vi "Script Execution.vi"() -> ()   [LabVIEW 2011]
uses:
  Classes/WorkorderHandler/Software/DataStructures/WorkorderHandler_ObjectReference.ctl
  <vilib>/Utility/miscctls.llb/LVRowAndColumnTypeDef.ctl
  Strict Type Controls/Settings Operation.ctl
  <vilib>/DAQmx/write.llb/DAQmx Write (Digital U32 1Chan 1Samp).vi
  <vilib>/DAQmx/create/channels.llb/DAQmx Create Channel (DO-Digital Output).vi
  <vilib>/DAQmx/miscellaneous.llb/DAQmx Fill In Error Info.vi
  <vilib>/Instr/_visa.llb/VISA Configure Serial Port (Instr).vi
panel:
  out "error out":errorcluster
  in  "error in (no error)":errorcluster
  out "Quit":bool
  in  "Heading":string="Regulator Test Bench With IEM Testing"
  in  "Edit":bool
  in  "Run":bool
  out "Order Number":string
  in  "Open":bool
  out "Bad Boards":u32
  out "Good Boards":u32
  out "result":bool=TRUE
  in  "Part Number":string
  out "Test Time":string
  in  "Result":i32(listbox)
  out "Regulator Voltage":dbl[](graph)
  out "DF Voltage":dbl[](graph)
  out "File Name":string
  out "Progress":u8(slide) scale=0.0..100.0
  # "App Designed For:"
  # "Web: www.jambhekar.com\nEmail: tushar@jambhekar.com\nCell: +919970168164"
  # "App Designed By:"
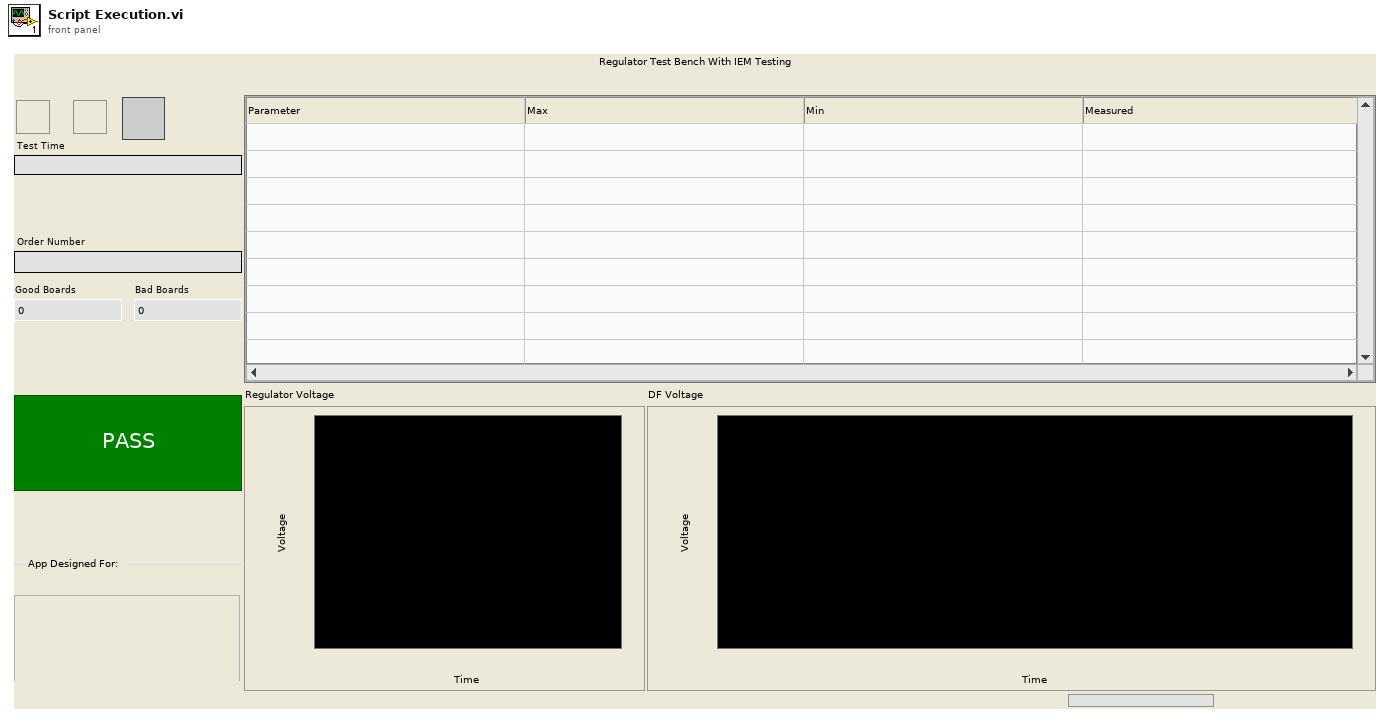
[diagram p1: front panel]
types:
  T1 = typedef "WorkorderHandler_ObjectReference.ctl" = refnum<k1>
  T2 = cluster{"Script":string[][], "Id":i32, "FailedOnce":bool, "Result":bool, "PassRef":refnum<file>, "FailRef":refnum<file>, "ScrName":string, "WORef":T1}
  T3 = enum32{"invalid app kind", "Development System", "Run Time System", "Student Edition", "Embedded LabVIEW", "Evaluation", "Custom"}
  T4 = typedef "Settings Operation.ctl" = enum8{"Get Value", "Set Value", "Read File", "Write File", "Write Stored Value"}
  T5 = typedef "LVRowAndColumnTypeDef.ctl" = cluster{"Row":i32, "Column":i32}
  T6 = enum32{"Invalid", "Standard", "Closed", "Hidden", "Minimized", "Maximized"}
  T7 = enum8{"Enabled", "Disabled", "Disabled and Grayed Out"}
  T8 = typedef "DispSettings.ctl" = cluster{"ShowDF":bool, "ShowPartNo":bool, "DF Pos":i32}
  T9 = cluster{"Port":refnum<visa-resource-name>, "baud rate":u32, "data bits":u16, "stop bits":u16, "parity":enum16{"None", "Odd", "Even", "Mark", "Space"}, "flow control":u16}
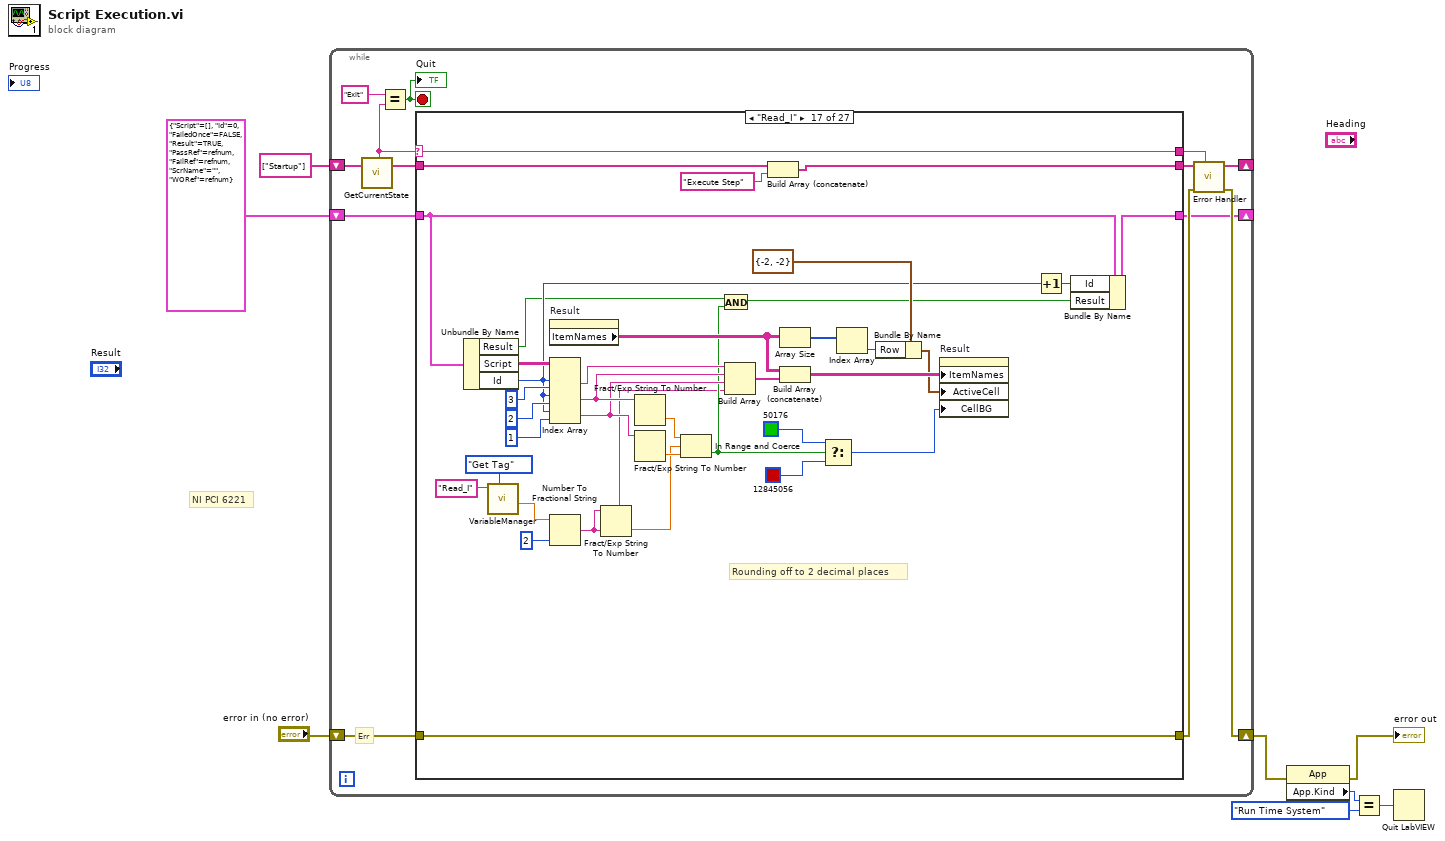
[diagram p0: block diagram]
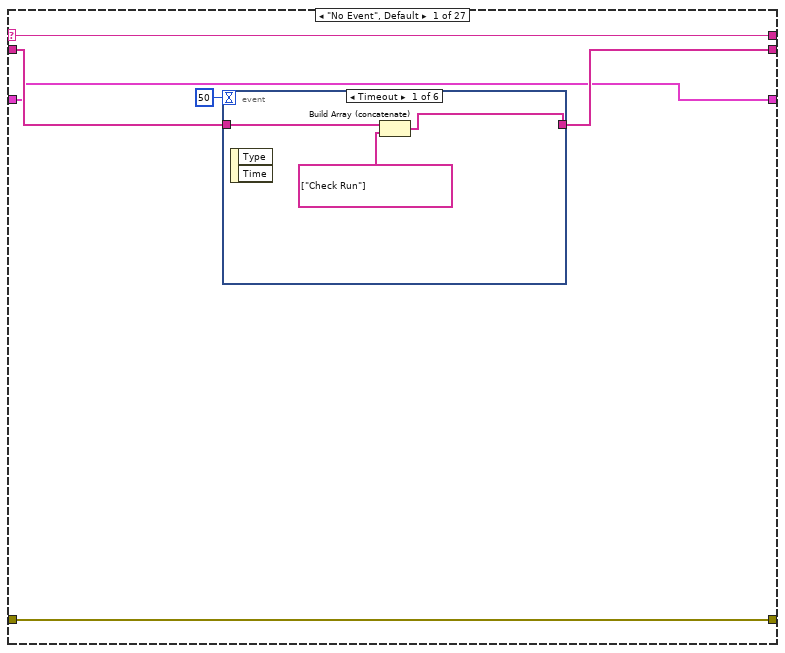
[diagram p2: hidden frame]
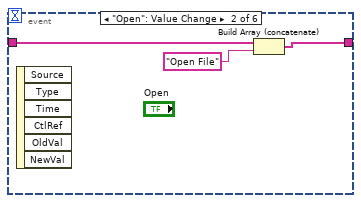
[diagram p3: hidden frame]
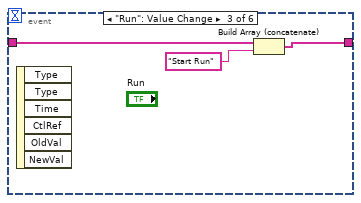
[diagram p4: hidden frame]
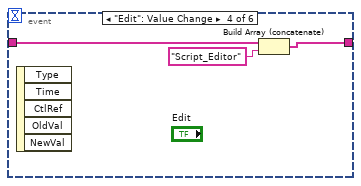
[diagram p5: hidden frame]
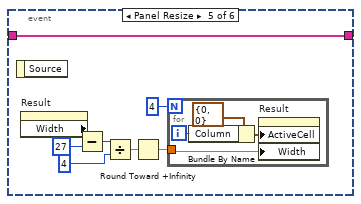
[diagram p6: hidden frame]
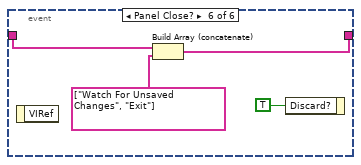
[diagram p7: hidden frame]
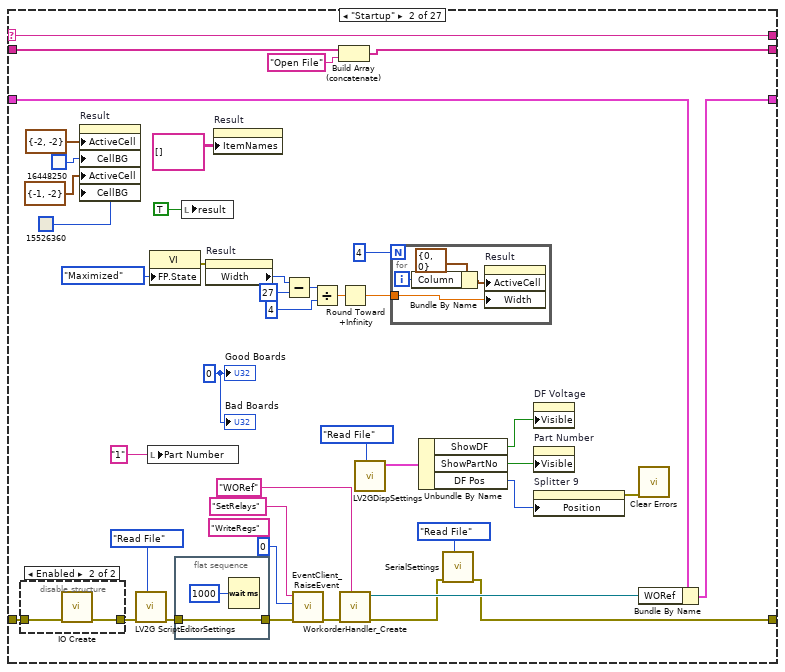
[diagram p8: hidden frame]
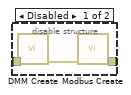
[diagram p9: hidden frame]
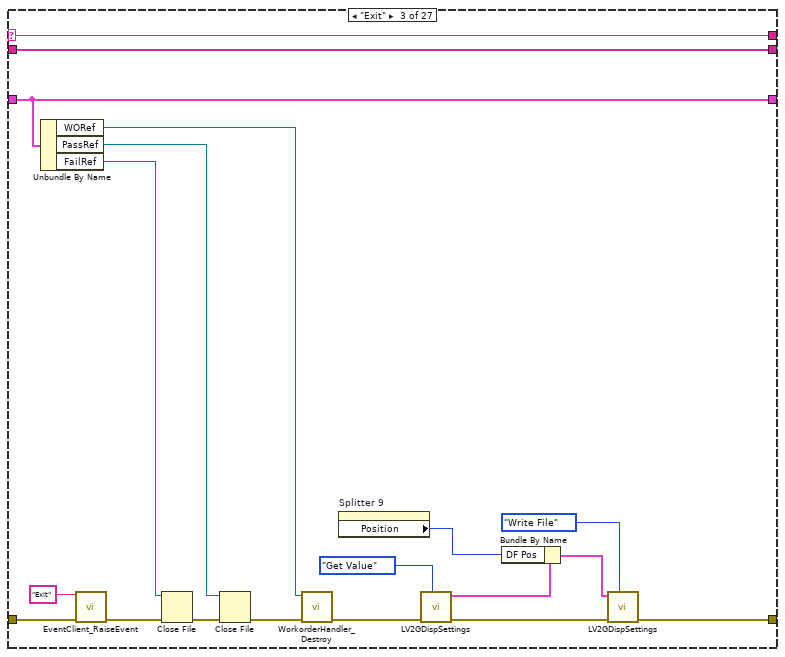
[diagram p10: hidden frame]
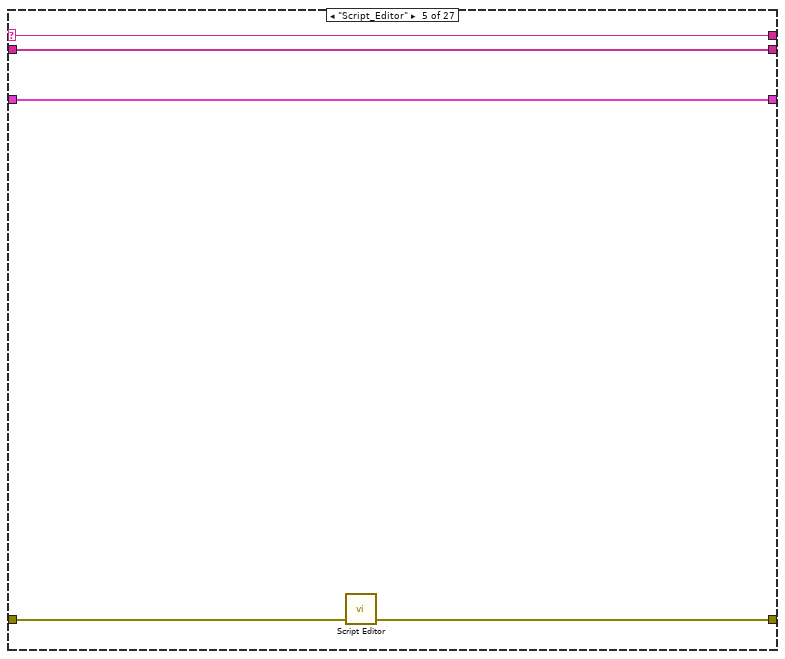
[diagram p12: hidden frame]
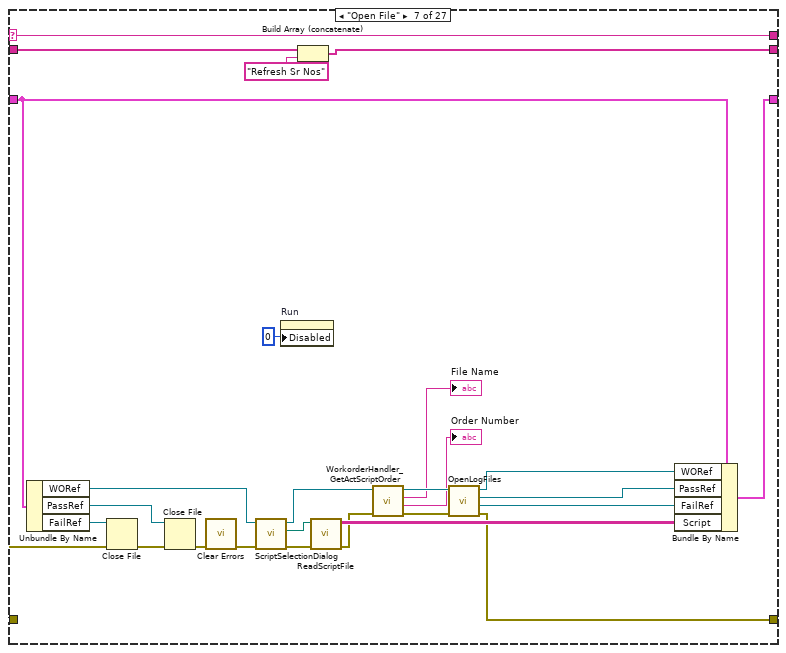
[diagram p14: hidden frame]
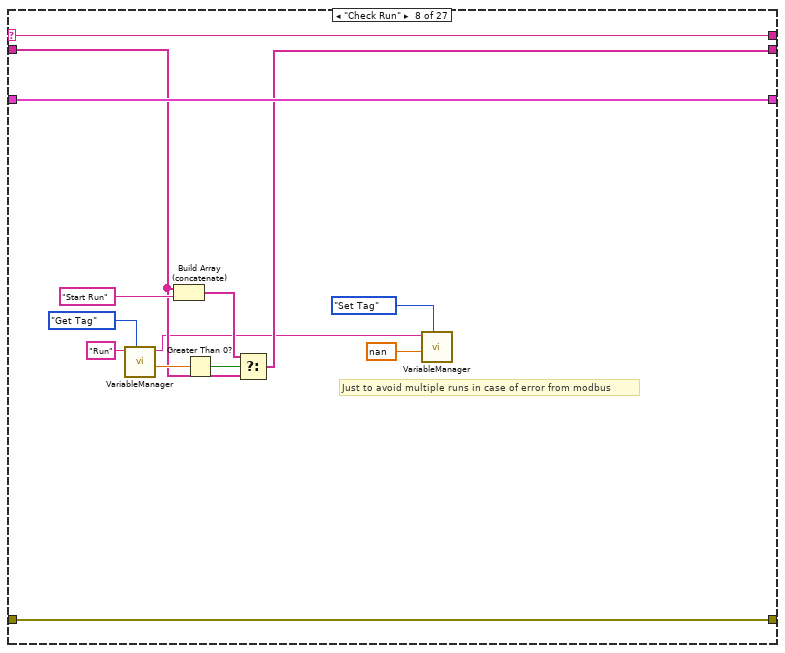
[diagram p15: hidden frame]
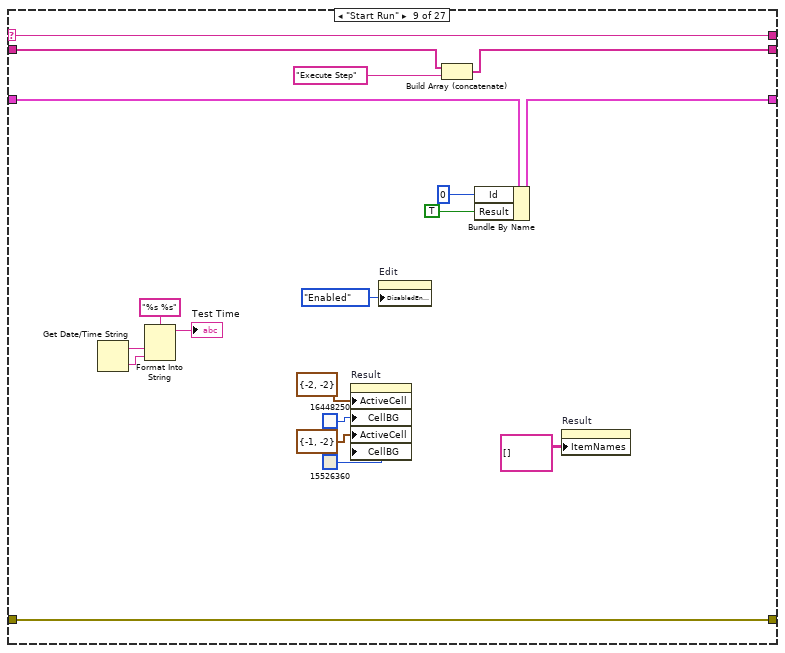
[diagram p16: hidden frame]
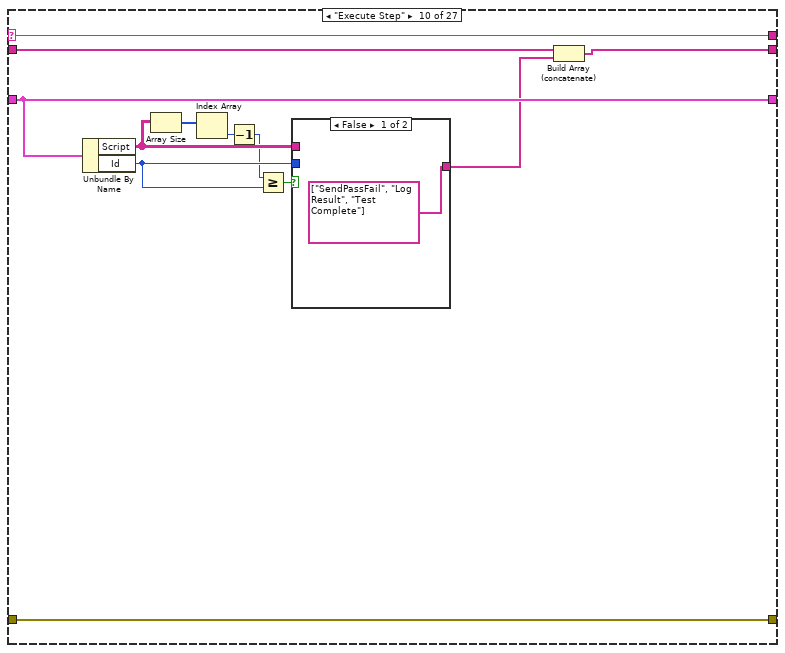
[diagram p17: hidden frame]
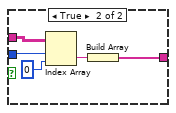
[diagram p18: hidden frame]
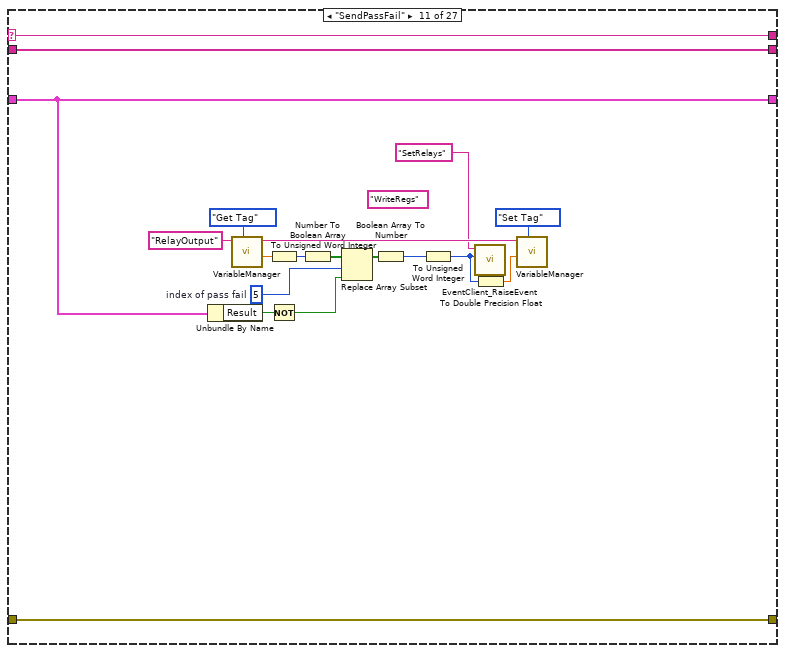
[diagram p19: hidden frame]
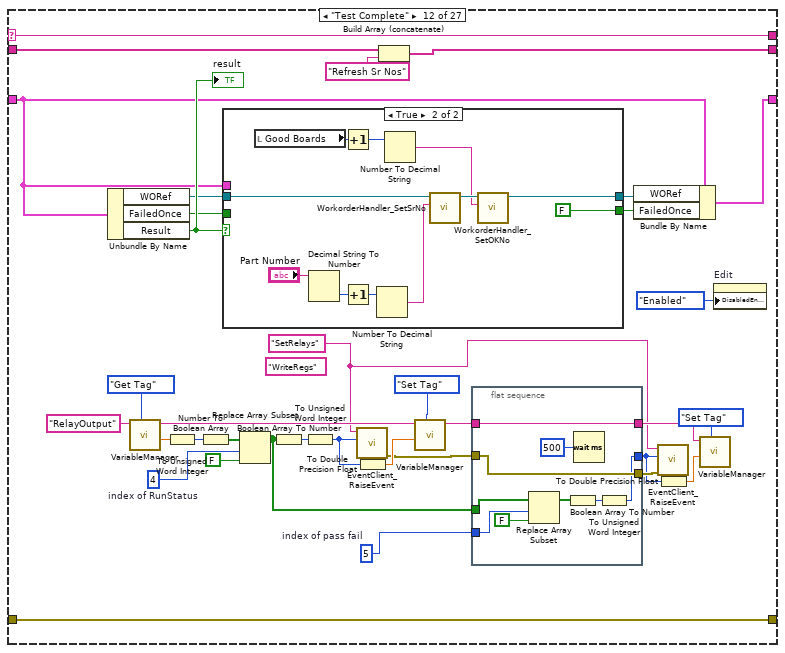
[diagram p20: hidden frame]
diagram:
  # "NI PCI 6221"
  n1 = while {
    shift-right: [w16] -> _
    shift-left: string[] ["Startup"] ("State Array Out") -> [w21]
    shift-right: [w13] -> w2
    shift-left: "error in (no error)" -> [w17]
    shift-right: [w10] -> _
    shift-left: T2 {"Script"=[], "Id"=0, "FailedOnce"=FALSE, "Result"=TRUE, "PassRef"=refnum, "FailRef"=refnum, "ScrName"="", "WORef"=refnum} ("Cluster") -> [w9]
    stop <- w18 stop-if-true
    # "Err"
    n2 = call "GetCurrentState.vi"("State Array In"=w21) -> ("Current State"=w11:string, "State Array Out"=w20:string[])  [unwired: 1 in, 16 out]
    n3 = Equal?(x="Exit", y=w11) -> (x = y?=w18:bool)
    "Quit" <- w18
    n4 = case shown="\"Read_I\"" w11 {
      selector: w11 -> [w27 w97 w126 w129 w136 w138 w167 w180 w199 w211 w236 w271 w329 w337 w374 w411 w448 w484 w521 w558 w572 w599 w628 w639 w655 w680 w684]
      tunnel: w20 -> [w23 w81 w127 w131 w135 w140 w142 w172 w190 w210 w235 w242 w328 w335 w372 w409 w446 w482 w519 w556 w570 w597 w626 w629 w646 w679 w683]
      tunnel: [w24 w80 w127 w131 w135 w140 w141 w171 w189 w209 w235 w241 w328 w335 w371 w408 w445 w481 w518 w555 w569 w596 w625 w629 w645 w679 w683] -> w15
      tunnel: [w26 w57 w114 w130 w132 w139 w144 w181 w200 w212 w237 w272 w314 w338 w375 w412 w449 w485 w522 w559 w573 w574 w610 w630 w648 w678 errorcluster {"status"=FALSE, "code"=0, "source"=""} ("error in (no error)")] -> w12
      tunnel: w17 -> [w26 w86 w125 w130 w133 w139 w158 w181 w200 w212 w237 w272 w315 w338 w375 w412 w449 w485 w522 w559 w573 w575 w611 w631 w649 w678 _]
      tunnel: [w27 w97 w126 w129 w136 w138 w167 w180 w199 w211 w236 w271 w329 w337 w374 w411 w448 w484 w521 w558 w572 w599 w628 w639 w655 w680 w684] -> w14
      tunnel: [w22 w67 w123 w128 w134 w137 w166 w175 w193 w206 w221 w266 w319 w336 w345 w382 w419 w458 w495 w532 w563 w590 w620 w636 w643 w677 w681] -> w10
      tunnel: w9 -> [w22 w68 w123 w128 w134 w137 w159 w175 w194 w206 w221 w267 w319 w336 w346 w383 w420 w459 w496 w533 w564 w591 w621 w636 w644 w677 w681]
      frame "No Event", Default {
        n5 = event shown="[0] Timeout" {
          selector: _ -> [_ _ _ _ _ _]
          dyn-events: _ -> [_ _ _ _ _ _]
          timeout: 50 -> [_ _ _ _ _ _]
          tunnel: w23 -> [w29 w33 w36 w39 w42 w54]
          tunnel: [w28 w32 w35 w38 w42 w52] -> w24
          event Timeout {
            n6 = event-data() -> ()  [unwired: 3 out]
            n7 = Build Array (concatenate)(w29, string[] ["Check Run"] ("State Array Out")) -> (w28:string[])
          }
          event "Open": Value Change {
            n8 = event-data() -> ()  [unwired: 7 out]
            n9 = Build Array (concatenate)(w33, "Open File" ("x")) -> (w32:string[])
          }
          event "Run": Value Change {
            n10 = event-data() -> ()  [unwired: 7 out]
            n11 = Build Array (concatenate)(w36, "Start Run" ("x")) -> (w35:string[])
          }
          event "Edit": Value Change {
            n12 = event-data() -> ()  [unwired: 6 out]
            n13 = Build Array (concatenate)(w39, "Script_Editor") -> (w38:string[])
          }
          event Panel Resize {
            n14 = event-data() -> ()  [unwired: 2 out]
            n15 = property on="Result" class="MCListbox (strict)"() -> ("Width"=w40:u32)  [unwired: 2 in, 2 out]
            n16 = Subtract(x=w40, y=u32 27) -> (x-y=w44:u32)
            n17 = Divide(x=w44, y=u32 4) -> (x/y=w46:dbl)
            n18 = Round Toward +Infinity(x=w46) -> (ceil(x): smallest int >= x=w47:dbl)
            n19 = for {
              N: 4 -> [_]
              tunnel: w47 -> [w48]
              i -> [w50]
              n20 = Bundle By Name(cluster=cluster{"Row":i32, "Column":i32} {"Row"=0, "Column"=0} ("Active Cell:Active Cell"), "Column"=w50) -> (w49:cluster{"Row":i32, "Column":i32})
              n21 = property on="Result" class="MCListbox (strict)"("ActiveCell"=w49, "Width"=w48) -> ()  [unwired: 2 in, 2 out]
            }
          }
          event Panel Close? {
            n22 = event-data() -> ()  [unwired: 2 out]
            n23 = Build Array (concatenate)(w54, string[] ["Watch For Unsaved Changes", "Exit"] ("State Array Out")) -> (w52:string[])
            n24 = event-data("Discard?"=TRUE) -> ()  [unwired: 1 in, 1 out]
          }
        }
      }
      frame "Startup" {
        w75 = u32 0 ("Good Boards")
        (unwired) "WriteRegs" ("Tag")
        n25 = disable-structure shown="Enabled" {
          disable-tunnel: w86 -> [w99 w102]
          disable-tunnel: [w98 w101] -> w85
          frame Disabled {
            n26 = call "DMM Create.vi"("error in (no error)"=w99) -> ("error out"=w100:errorcluster)  [unwired: 10 out]
            n27 = call "Modbus Create.vi"("error in (no error)"=w100) -> ("error out"=w98:errorcluster)  [unwired: 10 out]
          }
          frame Enabled {
            n28 = call "IO Create.vi"("error in (no error)"=w102) -> ("error out"=w101:errorcluster)  [unwired: 10 in]
          }
        }
        n29 = property on="Result" class="MCListbox (strict)"("ActiveCell"=T5 {"Row"=-2, "Column"=-2} ("Active Cell:Active Cell"), "CellBG"=u32 16448250, "ActiveCell"=T5 {"Row"=-1, "Column"=-2} ("Active Cell:Active Cell"), "CellBG"=u32 15526360 ("Color Box")) -> ()  [unwired: 2 in, 2 out]
        n30 = call "LV2G ScriptEditorSettings.vi"("Operation"=Settings_Operation."Read File", "error in (no error)"=w85) -> ("error out"=w77:errorcluster)  [unwired: 1 in, 8 out]
        n31 = local write "Part Number"("1" ("Part Number")) -> ()
        n32 = property class="VI"("FP.State"=T6."Maximized" ("Front Panel Window:State")) -> (error out=w87:errorcluster)  [unwired: 2 in, 1 out]
        n33 = flat-sequence {
          tunnel: [w103] -> w76
          tunnel: w77 -> [w103]
          frame #0 {
            n34 = Wait (ms)(milliseconds to wait=u32 1000) -> ()  [unwired: 1 out]
          }
        }
        n35 = local write "result"(TRUE ("result")) -> ()
        n36 = property on="Result" class="MCListbox (strict)"(error in=w87) -> ("Width"=w90:u32)  [unwired: 1 in, 2 out]
        n37 = property on="Result" class="MCListbox (strict)"("ItemNames"=string[][] [] ("Item Names")) -> ()  [unwired: 2 in, 2 out]
        n38 = Subtract(x=w90, y=u32 27) -> (x-y=w92:u32)
        n39 = call "EventClient_RaiseEvent.vi"("error in (no error)"=w76, "Data"=u16 0, "Event"="SetRelays" ("Tag")) -> ("error out"=w71:errorcluster)  [unwired: 1 in, 7 out]
        n40 = Divide(x=w92, y=u32 4) -> (x/y=w94:dbl)
        n41 = Build Array (concatenate)(w81, "Open File" ("String")) -> (w80:string[])
        n42 = Round Toward +Infinity(x=w94) -> (ceil(x): smallest int >= x=w95:dbl)
        n43 = call "WorkorderHandler_Create.vi"("object name (unnamed)"="WORef", "error in (no error)"=w71) -> ("error out"=w58:errorcluster, "reference"=w69:T1)  [unwired: 8 out]
        n44 = call "LV2GDispSettings.vi"("Operation"=Settings_Operation."Read File") -> ("DispSettings out"=w65:T8)  [unwired: 2 in, 8 out]
        n45 = for {
          N: 4 -> [_]
          tunnel: w95 -> [w105]
          i -> [w107]
          n46 = Bundle By Name(cluster=cluster{"Row":i32, "Column":i32} {"Row"=0, "Column"=0} ("Active Cell:Active Cell"), "Column"=w107) -> (w106:cluster{"Row":i32, "Column":i32})
          n47 = property on="Result" class="MCListbox (strict)"("ActiveCell"=w106, "Width"=w105) -> ()  [unwired: 2 in, 2 out]
        }
        n48 = Unbundle By Name(w65) -> ("ShowDF"=w63:bool, "ShowPartNo"=w62:bool, "DF Pos"=w64:i32)
        n49 = call "SerialSettings.vi"("Operation"=Settings_Operation."Read File", "error in (no error)"=w58) -> ("error out"=w57:errorcluster)  [unwired: 8 in, 1 out]
        n50 = property on="DF Voltage" class="WFGraph (strict)"("Visible"=w63) -> ()  [unwired: 2 in, 2 out]
        n51 = property on="Part Number" class="Str"("Visible"=w62) -> ()  [unwired: 2 in, 2 out]
        n52 = property on="Splitter 9" class="Splitter"("Position"=w64) -> (error out=w61:errorcluster)  [unwired: 2 in, 1 out]
        n53 = call <vilib>:"Clear Errors.vi"("error in (no error)"=w61) -> ()  [unwired: 7 out]
        n54 = Bundle By Name(cluster=w68, "WORef"=w69) -> (w67:T2)
        "Good Boards" <- w75
        "Bad Boards" <- w75
      }
      frame "Exit" {
        n55 = Unbundle By Name(w123) -> ("WORef"=w117:T1, "PassRef"=w119:refnum<file>, "FailRef"=w120:refnum<file>)
        n56 = call "EventClient_RaiseEvent.vi"("error in (no error)"=w125, "Event"="Exit" ("x")) -> ("error out"=w122:errorcluster)  [unwired: 2 in, 7 out]
        n57 = Close File(refnum=w120, error in=w122) -> (error out=w121:errorcluster)  [unwired: 1 out]
        n58 = Close File(refnum=w119, error in=w121) -> (error out=w118:errorcluster)  [unwired: 1 out]
        n59 = call "WorkorderHandler_Destroy.vi"("error in (no error)"=w118, "reference"=w117) -> ("error out"=w116:errorcluster)  [unwired: 9 out]
        n60 = property on="Splitter 9" class="Splitter"() -> ("Position"=w109:i32)  [unwired: 2 in, 2 out]
        n61 = call "LV2GDispSettings.vi"("Operation"=Settings_Operation."Get Value", "error in (no error)"=w116) -> ("error out"=w115:errorcluster, "DispSettings out"=w111:T8)  [unwired: 1 in, 7 out]
        n62 = Bundle By Name(cluster=w111, "DF Pos"=w109) -> (w110:T8)
        n63 = call "LV2GDispSettings.vi"("Operation"=Settings_Operation."Write File", "error in (no error)"=w115, "DispSettings"=w110) -> ("error out"=w114:errorcluster)  [unwired: 8 out]
      }
      frame "---------------Below are UI Events---------------" {
      }
      frame "Script_Editor" {
        n64 = call "Script Editor.vi"("error in (no error)"=w133) -> ("error out"=w132:errorcluster)  [unwired: 4 in]
      }
      frame "---------------Below are Subroutine states---------------" {
      }
      frame "Open File" {
        n65 = Unbundle By Name(w159) -> ("WORef"=w155:T1, "PassRef"=w161:refnum<file>, "FailRef"=w160:refnum<file>)
        n66 = Close File(refnum=w160, error in=w158) -> (error out=w162:errorcluster)  [unwired: 1 out]
        n67 = Close File(refnum=w161, error in=w162) -> (error out=w157:errorcluster)  [unwired: 1 out]
        n68 = call <vilib>:"Clear Errors.vi"("error in (no error)"=w157) -> ("error out"=w156:errorcluster)  [unwired: 6 out]
        n69 = call "ScriptSelectionDialog.vi"("error in (no error)"=w156, "WORef"=w155) -> ("error out"=w163:errorcluster, "Path"=w154:path, "WORef Out"=w151:T1)  [unwired: 7 out]
        n70 = property on="Run" class="Bool"("Disabled"=u8 0) -> ()  [unwired: 2 in, 2 out]
        n71 = Build Array (concatenate)(w142, "Refresh Sr Nos" ("x")) -> (w141:string[])
        n72 = call "ReadScriptFile.vi"("error in (no error)"=w163, "File"=w154) -> ("error out"=w149:errorcluster, "Script"=w164:string[][])  [unwired: 1 in, 7 out]
        n73 = call "WorkorderHandler_GetActScriptOrder.vi"("error in (no error)"=w149, "reference"=w151) -> ("error out"=w148:errorcluster, "Order"=→"Order Number":string, "Script"=→"File Name":string, "duplicate reference"=w150:T1)  [unwired: 6 out]
        n74 = call "OpenLogFiles.vi"("error in (no error)"=w148, "WORef"=w150) -> ("error out"=w144:errorcluster, "FailRef"=w153:refnum<file>, "PassRef"=w152:refnum<file>, "WORef Out"=w145:T1)  [unwired: 6 out]
        n75 = Bundle By Name(cluster=w159, "WORef"=w145, "PassRef"=w152, "FailRef"=w153, "Script"=w164) -> (w166:T2)
      }
      frame "Check Run" {
        # "Just to avoid multiple runs in case of error from modbus"
        n76 = call "VariableManager.vi"("Operation"=enum16{"Get Tag", "Set Tag"}."Get Tag", "Tag"="Run") -> ("Value out"=w177:dbl, "Tag Out"=w169:string)  [unwired: 1 in, 7 out]
        n77 = Build Array (concatenate)(w172, "Start Run" ("x")) -> (w173:string[])
        n78 = Greater Than 0?(x=w177) -> (x > 0?=w176:bool)
        n79 = Select(t=w173, s=w176, f=w172) -> (s? t:f=w171:string[])
        n80 = call "VariableManager.vi"("Operation"=enum16{"Get Tag", "Set Tag"}."Set Tag", "Value"=nan, "Tag"=w169) -> ()  [unwired: 9 out]
      }
      frame "Start Run" {
        n81 = Get Date/Time String() -> (date string=w198:string, time string=w197:string)  [unwired: 3 out]
        n82 = Format Into String(format string="%s %s", w198, w197) -> (resulting string=→"Test Time":string)  [unwired: 2 in, 1 out]
        n83 = property on="Result" class="MCListbox (strict)"("ActiveCell"=T5 {"Row"=-2, "Column"=-2} ("Active Cell:Active Cell"), "CellBG"=u32 16448250, "ActiveCell"=T5 {"Row"=-1, "Column"=-2} ("Active Cell:Active Cell"), "CellBG"=u32 15526360 ("Color Box")) -> ()  [unwired: 2 in, 2 out]
        n84 = property on="Edit" class="Bool"("DisabledEnum"=T7."Enabled" ("Disabled")) -> ()  [unwired: 2 in, 2 out]
        n85 = Build Array (concatenate)(w190, "Execute Step" ("x")) -> (w189:string[])
        n86 = Bundle By Name(cluster=w194, "Id"=0, "Result"=TRUE) -> (w193:T2)
        n87 = property on="Result" class="MCListbox (strict)"("ItemNames"=string[][] [] ("Item Names")) -> ()  [unwired: 2 in, 2 out]
      }
      frame "Execute Step" {
        n88 = Unbundle By Name(w206) -> ("Script"=w204:string[][], "Id"=w203:i32)
        n89 = Array Size(array=w204) -> (size(s)=w208:i32[])
        n90 = Index Array(array=w208) -> (element=w207:i32)  [unwired: 1 in]
        n91 = Decrement(x=w207) -> (x-1=w201:i32)
        n92 = Greater Or Equal?(x=w201, y=w203) -> (x >= y?=w205:bool)
        n93 = case shown="False" w205 {
          tunnel: w204 -> [_ w218]
          tunnel: w203 -> [_ w217]
          tunnel: [string[] ["SendPassFail", "Log Result", "Test Complete"] ("State Array Out") w214] -> w202
          frame False {
          }
          frame True {
            n94 = Index Array(array=w218, index (row)=w217, index (col)=0 ("disabled index (col)")) -> (element=w215:string)
            n95 = Build Array(w215) -> (w214:string[])
          }
        }
        n96 = Build Array (concatenate)(w210, w202) -> (w209:string[])
      }
      frame "SendPassFail" {
        w227 = 5  # index of pass fail
        (unwired) "WriteRegs" ("Tag")
        n97 = Unbundle By Name(w221) -> ("Result"=w220:bool)
        n98 = call "VariableManager.vi"("Operation"=enum16{"Get Tag", "Set Tag"}."Get Tag", "Tag"="RelayOutput") -> ("Value out"=w232:dbl, "Tag Out"=w222:string)  [unwired: 1 in, 7 out]
        n99 = To Unsigned Word Integer(number=w232) -> (unsigned 16bit integer=w231:u16)
        n100 = Not(x=w220) -> (.not. x?=w226:bool)
        n101 = Number To Boolean Array(number=w231) -> (Boolean array=w230:bool[])
        n102 = Replace Array Subset(array=w230, new element=w226, index=w227) -> (w229:bool[])
        n103 = Boolean Array To Number(Boolean array=w229) -> (number=w228:u32)
        n104 = To Unsigned Word Integer(number=w228) -> (unsigned 16bit integer=w224:u16)
        n105 = call "EventClient_RaiseEvent.vi"("Data"=w224, "Event"="SetRelays" ("Tag")) -> ()  [unwired: 2 in, 8 out]
        n106 = To Double Precision Float(number=w224) -> (double precision float=w223:dbl)
        n107 = call "VariableManager.vi"("Operation"=enum16{"Get Tag", "Set Tag"}."Set Tag", "Value"=w223, "Tag"=w222) -> ()  [unwired: 9 out]
      }
      frame "Test Complete" {
        w238 = "SetRelays" ("Tag")
        w252 = 5  # index of pass fail
        w259 = 4  # index of RunStatus
        (unwired) "WriteRegs" ("Tag")
        n108 = Unbundle By Name(w267) -> ("WORef"=w244:T1, "FailedOnce"=w268:bool, "Result"=w269:bool)
        "result" <- w269
        n109 = call "VariableManager.vi"("Operation"=enum16{"Get Tag", "Set Tag"}."Get Tag", "Tag"="RelayOutput") -> ("Value out"=w263:dbl, "Tag Out"=w256:string)  [unwired: 1 in, 7 out]
        n110 = To Unsigned Word Integer(number=w263) -> (unsigned 16bit integer=w262:u16)
        n111 = Number To Boolean Array(number=w262) -> (Boolean array=w261:bool[])
        n112 = case shown="True" w269 {
          tunnel: w267 -> [_ _]
          tunnel: [w285 FALSE] -> w270
          tunnel: w268 -> [w284 _]
          tunnel: w244 -> [w283 w298]
          tunnel: [w282 w294] -> w243
          frame False {
            n113 = case shown="True" w284 {
              tunnel: [TRUE FALSE] -> w285
              tunnel: w283 -> [w286 w291]
              tunnel: [w286 w288] -> w282
              frame False {
              }
              frame True {
                n114 = local read "Bad Boards"() -> (w293:u32)
                n115 = Increment(x=w293) -> (x+1=w290:u32)
                n116 = Number To Decimal String(number=w290) -> (decimal integer string=w289:string)  [unwired: 1 out]
                n117 = call "WorkorderHandler_SetBadNo.vi"("BadNo"=w289, "reference"=w291) -> ("duplicate reference"=w288:T1)  [unwired: 1 in, 8 out]
              }
            }
          }
          frame True {
            n118 = local read "Good Boards"() -> (w301:u32)
            n119 = Decimal String To Number(string="Part Number") -> (number=w304:i32)  [unwired: 3 out]
            n120 = Increment(x=w301) -> (x+1=w296:u32)
            n121 = Increment(x=w304) -> (x+1=w303:i32)
            n122 = Number To Decimal String(number=w303) -> (decimal integer string=w299:string)  [unwired: 1 out]
            n123 = Number To Decimal String(number=w296) -> (decimal integer string=w295:string)  [unwired: 1 out]
            n124 = call "WorkorderHandler_SetSrNo.vi"("SrNo"=w299, "reference"=w298) -> ("duplicate reference"=w297:T1)  [unwired: 1 in, 8 out]
            n125 = call "WorkorderHandler_SetOKNo.vi"("OKNo"=w295, "reference"=w297) -> ("duplicate reference"=w294:T1)  [unwired: 1 in, 8 out]
          }
        }
        n126 = Replace Array Subset(array=w261, new element=FALSE ("new element/subarray"), index=w259) -> (w253:bool[])
        n127 = Boolean Array To Number(Boolean array=w253) -> (number=w260:u32)
        n128 = To Unsigned Word Integer(number=w260) -> (unsigned 16bit integer=w254:u16)
        n129 = call "EventClient_RaiseEvent.vi"("Data"=w254, "Event"=w238) -> ("error out"=w249:errorcluster)  [unwired: 2 in, 7 out]
        n130 = To Double Precision Float(number=w254) -> (double precision float=w257:dbl)
        n131 = Build Array (concatenate)(w242, "Refresh Sr Nos" ("x")) -> (w241:string[])
        n132 = call "VariableManager.vi"("Operation"=enum16{"Get Tag", "Set Tag"}."Set Tag", "Value"=w257, "Tag"=w256) -> ("Tag Out"=w245:string)  [unwired: 8 out]
        n133 = flat-sequence {
          tunnel: w253 -> [w280]
          tunnel: w252 -> [w279]
          tunnel: w249 -> [w276]
          tunnel: [w276] -> w248
          tunnel: [w275] -> w247
          tunnel: [w274] -> w246
          tunnel: w245 -> [w274]
          frame #0 {
            n134 = Replace Array Subset(array=w280, new element=FALSE ("new element/subarray"), index=w279) -> (w277:bool[])
            n135 = Boolean Array To Number(Boolean array=w277) -> (number=w278:u32)
            n136 = Wait (ms)(milliseconds to wait=u32 500) -> ()  [unwired: 1 out]
            n137 = To Unsigned Word Integer(number=w278) -> (unsigned 16bit integer=w275:u16)
          }
        }
        n138 = Bundle By Name(cluster=w267, "WORef"=w243, "FailedOnce"=w270) -> (w266:T2)
        n139 = call "EventClient_RaiseEvent.vi"("error in (no error)"=w248, "Data"=w247, "Event"=w238) -> ()  [unwired: 1 in, 8 out]
        n140 = To Double Precision Float(number=w247) -> (double precision float=w251:dbl)
        n141 = call "VariableManager.vi"("Operation"=enum16{"Get Tag", "Set Tag"}."Set Tag", "Value"=w251, "Tag"=w246) -> ()  [unwired: 9 out]
        n142 = property on="Edit" class="Bool"("DisabledEnum"=T7."Enabled" ("Disabled")) -> ()  [unwired: 2 in, 2 out]
      }
      frame "Log Result" {
        n143 = local read "Good Boards"() -> (w309:u32)
        n144 = local read "Bad Boards"() -> (w308:u32)
        n145 = Unbundle By Name(w319) -> ("PassRef"=w318:refnum<file>, "Result"=w310:bool, "FailRef"=w317:refnum<file>, "FailedOnce"=w311:bool)
        n146 = Or(x=w310, y=w311) -> (x .or. y?=w312:bool)
        n147 = Select(t=w318, s=w310, f=w317) -> (s? t:f=w316:refnum<file>)
        n148 = Select(t=w309, s=w310, f=w308) -> (s? t:f=w307:u32)
        n149 = Increment(x=w307) -> (x+1=w305:u32)
        n150 = Number To Decimal String(number=w305) -> (decimal integer string=w306:string)  [unwired: 1 out]
        n151 = local read "Test Time"() -> (w313:string)
        n152 = property on="Result" class="MCListbox (strict)"() -> ("ItemNames"=w327:string[][])  [unwired: 2 in, 2 out]
        n153 = Index Array(array=w327, index (col)=3 ("disabled index (col)")) -> (element=w321:string[])  [unwired: 1 in]
        n154 = Build Array (concatenate)(w306, w313, w321) -> (w320:string[])
        n155 = Array To Spreadsheet String(array=w320, 3:"%s" ("format string")) -> (spreadsheet string=w323:string)  [unwired: 1 out]
        n156 = Concatenate Strings(w323, "\r\n") -> (w322:string)
        n157 = case shown="True" w312 {
          tunnel: w322 -> [_ w334]
          tunnel: w316 -> [_ w333]
          tunnel: w315 -> [w330 w332]
          tunnel: [w330 w331] -> w314
          frame False {
          }
          frame True {
            n158 = Write to Text File(file (use dialog)=w333, text=w334, error in=w332) -> (error out=w331:errorcluster)  [unwired: 3 out]
          }
        }
      }
      frame "---------------Below are Step states---------------" {
      }
      frame "Read DMM" {
        # "Rounding off to 2 decimal places"
        n159 = Unbundle By Name(w346) -> ("Result"=w343:bool, "Script"=w370:string[][], "Id"=w347:i32)
        n160 = call "VariableManager.vi"("Operation"=enum16{"Get Tag", "Set Tag"}."Get Tag", "Tag"="DMM") -> ("Value out"=w359:dbl)  [unwired: 1 in, 8 out]
        n161 = property on="Result" class="MCListbox (strict)"() -> ("ItemNames"=w356:string[][])  [unwired: 2 in, 2 out]
        n162 = Index Array(array=w370, index (row) #1=w347, index (col) #1=3 ("disabled index (col)"), index (row) #2=w347, index (col) #2=2 ("disabled index (col)"), index (row) #3=w347, index (col) #3=1 ("disabled index (col)")) -> (element #1=w365:string, element #2=w363:string, element #3=w362:string)
        n163 = Number To Fractional String(number=w359, precision (6)=i16 2) -> (F-format string=w340:string)  [unwired: 2 out]
        n164 = Fract/Exp String To Number(string=w340) -> (number=w339:dbl)  [unwired: 4 out]
        n165 = Fract/Exp String To Number(string=w363) -> (number=w361:dbl)  [unwired: 4 out]
        n166 = Fract/Exp String To Number(string=w362) -> (number=w360:dbl)  [unwired: 4 out]
        n167 = In Range and Coerce(upper limit=w361, x=w339, lower limit=w360) -> (In Range?=w344:bool)  [unwired: 1 out]
        n168 = And(x=w343, y=w344) -> (x .and. y?=w342:bool)
        n169 = Build Array(w365, w363, w362, w340) -> (w358:string[])
        n170 = Build Array (concatenate)(w372, "Execute Step" ("x")) -> (w371:string[])
        n171 = Array Size(array=w356) -> (size(s)=w355:i32[])
        n172 = Build Array (concatenate)(w356, w358) -> (w357:string[][])
        n173 = Select(t=u32 50176, s=w344, f=u32 12845056) -> (s? t:f=w349:u32)
        n174 = Index Array(array=w355) -> (element=w353:i32)  [unwired: 1 in]
        n175 = Bundle By Name(cluster=T5 {"Row"=-2, "Column"=-2} ("Active Cell:Active Cell"), "Row"=w353) -> (w352:T5)
        n176 = property on="Result" class="MCListbox (strict)"("ItemNames"=w357, "ActiveCell"=w352, "CellBG"=w349) -> ()  [unwired: 2 in, 2 out]
        n177 = Increment(x=w347) -> (x+1=w348:i32)
        n178 = Bundle By Name(cluster=w346, "Id"=w348, "Result"=w342) -> (w345:T2)
      }
      frame "Read_V" {
        # "Rounding off to 2 decimal places"
        n179 = Unbundle By Name(w383) -> ("Result"=w380:bool, "Script"=w407:string[][], "Id"=w384:i32)
        n180 = call "VariableManager.vi"("Operation"=enum16{"Get Tag", "Set Tag"}."Get Tag", "Tag"="Read_V") -> ("Value out"=w396:dbl)  [unwired: 1 in, 8 out]
        n181 = property on="Result" class="MCListbox (strict)"() -> ("ItemNames"=w393:string[][])  [unwired: 2 in, 2 out]
        n182 = Index Array(array=w407, index (row) #1=w384, index (col) #1=3 ("disabled index (col)"), index (row) #2=w384, index (col) #2=2 ("disabled index (col)"), index (row) #3=w384, index (col) #3=1 ("disabled index (col)")) -> (element #1=w402:string, element #2=w400:string, element #3=w399:string)
        n183 = Number To Fractional String(number=w396, precision (6)=i16 2) -> (F-format string=w377:string)  [unwired: 2 out]
        n184 = Fract/Exp String To Number(string=w377) -> (number=w376:dbl)  [unwired: 4 out]
        n185 = Fract/Exp String To Number(string=w400) -> (number=w398:dbl)  [unwired: 4 out]
        n186 = Fract/Exp String To Number(string=w399) -> (number=w397:dbl)  [unwired: 4 out]
        n187 = In Range and Coerce(upper limit=w398, x=w376, lower limit=w397) -> (In Range?=w381:bool)  [unwired: 1 out]
        n188 = And(x=w380, y=w381) -> (x .and. y?=w379:bool)
        n189 = Build Array(w402, w400, w399, w377) -> (w395:string[])
        n190 = Build Array (concatenate)(w409, "Execute Step" ("x")) -> (w408:string[])
        n191 = Array Size(array=w393) -> (size(s)=w392:i32[])
        n192 = Build Array (concatenate)(w393, w395) -> (w394:string[][])
        n193 = Select(t=u32 50176, s=w381, f=u32 12845056) -> (s? t:f=w386:u32)
        n194 = Index Array(array=w392) -> (element=w390:i32)  [unwired: 1 in]
        n195 = Bundle By Name(cluster=T5 {"Row"=-2, "Column"=-2} ("Active Cell:Active Cell"), "Row"=w390) -> (w389:T5)
        n196 = property on="Result" class="MCListbox (strict)"("ItemNames"=w394, "ActiveCell"=w389, "CellBG"=w386) -> ()  [unwired: 2 in, 2 out]
        n197 = Increment(x=w384) -> (x+1=w385:i32)
        n198 = Bundle By Name(cluster=w383, "Id"=w385, "Result"=w379) -> (w382:T2)
      }
      frame "Read_I" {
        # "Rounding off to 2 decimal places"
        n199 = Unbundle By Name(w420) -> ("Result"=w417:bool, "Script"=w444:string[][], "Id"=w421:i32)
        n200 = call "VariableManager.vi"("Operation"=enum16{"Get Tag", "Set Tag"}."Get Tag", "Tag"="Read_I") -> ("Value out"=w433:dbl)  [unwired: 1 in, 8 out]
        n201 = property on="Result" class="MCListbox (strict)"() -> ("ItemNames"=w430:string[][])  [unwired: 2 in, 2 out]
        n202 = Index Array(array=w444, index (row) #1=w421, index (col) #1=3 ("disabled index (col)"), index (row) #2=w421, index (col) #2=2 ("disabled index (col)"), index (row) #3=w421, index (col) #3=1 ("disabled index (col)")) -> (element #1=w439:string, element #2=w437:string, element #3=w436:string)
        n203 = Number To Fractional String(number=w433, precision (6)=i16 2) -> (F-format string=w414:string)  [unwired: 2 out]
        n204 = Fract/Exp String To Number(string=w414) -> (number=w413:dbl)  [unwired: 4 out]
        n205 = Fract/Exp String To Number(string=w437) -> (number=w435:dbl)  [unwired: 4 out]
        n206 = Fract/Exp String To Number(string=w436) -> (number=w434:dbl)  [unwired: 4 out]
        n207 = In Range and Coerce(upper limit=w435, x=w413, lower limit=w434) -> (In Range?=w418:bool)  [unwired: 1 out]
        n208 = And(x=w417, y=w418) -> (x .and. y?=w416:bool)
        n209 = Build Array(w439, w437, w436, w414) -> (w432:string[])
        n210 = Build Array (concatenate)(w446, "Execute Step" ("x")) -> (w445:string[])
        n211 = Array Size(array=w430) -> (size(s)=w429:i32[])
        n212 = Build Array (concatenate)(w430, w432) -> (w431:string[][])
        n213 = Select(t=u32 50176, s=w418, f=u32 12845056) -> (s? t:f=w423:u32)
        n214 = Index Array(array=w429) -> (element=w427:i32)  [unwired: 1 in]
        n215 = Bundle By Name(cluster=T5 {"Row"=-2, "Column"=-2} ("Active Cell:Active Cell"), "Row"=w427) -> (w426:T5)
        n216 = property on="Result" class="MCListbox (strict)"("ItemNames"=w431, "ActiveCell"=w426, "CellBG"=w423) -> ()  [unwired: 2 in, 2 out]
        n217 = Increment(x=w421) -> (x+1=w422:i32)
        n218 = Bundle By Name(cluster=w420, "Id"=w422, "Result"=w416) -> (w419:T2)
      }
      frame "Read Reg Freq" {
        # "Rounding off to 2 decimal places"
        n219 = Unbundle By Name(w459) -> ("Result"=w455:bool, "Script"=w480:string[][], "Id"=w460:i32)
        n220 = call "ReadFreqVoltage.vi"("channel"=tag "Dev1/ai0") -> ("frequency"=w451:dbl)  [unwired: 1 in, 9 out]
        n221 = property on="Result" class="MCListbox (strict)"() -> ("ItemNames"=w469:string[][])  [unwired: 2 in, 2 out]
        n222 = Index Array(array=w480, index (row) #1=w460, index (col) #1=3 ("disabled index (col)"), index (row) #2=w460, index (col) #2=2 ("disabled index (col)"), index (row) #3=w460, index (col) #3=1 ("disabled index (col)")) -> (element #1=w476:string, element #2=w475:string, element #3=w474:string)
        n223 = Number To Fractional String(number=w451, precision (6)=i16 2) -> (F-format string=w452:string)  [unwired: 2 out]
        n224 = Fract/Exp String To Number(string=w452) -> (number=w450:dbl)  [unwired: 4 out]
        n225 = Fract/Exp String To Number(string=w475) -> (number=w473:dbl)  [unwired: 4 out]
        n226 = Fract/Exp String To Number(string=w474) -> (number=w472:dbl)  [unwired: 4 out]
        n227 = In Range and Coerce(upper limit=w473, x=w450, lower limit=w472) -> (In Range?=w457:bool)  [unwired: 1 out]
        n228 = Build Array(w476, w475, w474, w452) -> (w471:string[])
        n229 = And(x=w455, y=w457) -> (x .and. y?=w454:bool)
        n230 = Build Array (concatenate)(w482, "Execute Step" ("x")) -> (w481:string[])
        n231 = Array Size(array=w469) -> (size(s)=w468:i32[])
        n232 = Build Array (concatenate)(w469, w471) -> (w470:string[][])
        n233 = Select(t=u32 50176, s=w457, f=u32 12845056) -> (s? t:f=w462:u32)
        n234 = Index Array(array=w468) -> (element=w466:i32)  [unwired: 1 in]
        n235 = Bundle By Name(cluster=T5 {"Row"=-2, "Column"=-2} ("Active Cell:Active Cell"), "Row"=w466) -> (w465:T5)
        n236 = property on="Result" class="MCListbox (strict)"("ItemNames"=w470, "ActiveCell"=w465, "CellBG"=w462) -> ()  [unwired: 2 in, 2 out]
        n237 = Increment(x=w460) -> (x+1=w461:i32)
        n238 = Bundle By Name(cluster=w459, "Id"=w461, "Result"=w454) -> (w458:T2)
      }
      frame "Read Reg V" {
        # "Rounding off to 2 decimal places"
        n239 = Unbundle By Name(w496) -> ("Result"=w490:bool, "Script"=w517:string[][], "Id"=w497:i32)
        n240 = call "ReadFreqVoltage.vi"("channel"=tag "Dev1/ai0") -> ("Waveform"=→"Regulator Voltage":dbl[], "Avg"=w492:dbl)  [unwired: 1 in, 8 out]
        n241 = property on="Result" class="MCListbox (strict)"() -> ("ItemNames"=w506:string[][])  [unwired: 2 in, 2 out]
        n242 = Index Array(array=w517, index (row) #1=w497, index (col) #1=3 ("disabled index (col)"), index (row) #2=w497, index (col) #2=2 ("disabled index (col)"), index (row) #3=w497, index (col) #3=1 ("disabled index (col)")) -> (element #1=w513:string, element #2=w512:string, element #3=w511:string)
        n243 = Number To Fractional String(number=w492, precision (6)=i16 2) -> (F-format string=w487:string)  [unwired: 2 out]
        n244 = Fract/Exp String To Number(string=w487) -> (number=w486:dbl)  [unwired: 4 out]
        n245 = Fract/Exp String To Number(string=w512) -> (number=w510:dbl)  [unwired: 4 out]
        n246 = Fract/Exp String To Number(string=w511) -> (number=w509:dbl)  [unwired: 4 out]
        n247 = In Range and Coerce(upper limit=w510, x=w486, lower limit=w509) -> (In Range?=w494:bool)  [unwired: 1 out]
        n248 = Build Array(w513, w512, w511, w487) -> (w508:string[])
        n249 = And(x=w490, y=w494) -> (x .and. y?=w489:bool)
        n250 = Build Array (concatenate)(w519, "Execute Step" ("x")) -> (w518:string[])
        n251 = Array Size(array=w506) -> (size(s)=w505:i32[])
        n252 = Build Array (concatenate)(w506, w508) -> (w507:string[][])
        n253 = Select(t=u32 50176, s=w494, f=u32 12845056) -> (s? t:f=w499:u32)
        n254 = Index Array(array=w505) -> (element=w503:i32)  [unwired: 1 in]
        n255 = Bundle By Name(cluster=T5 {"Row"=-2, "Column"=-2} ("Active Cell:Active Cell"), "Row"=w503) -> (w502:T5)
        n256 = property on="Result" class="MCListbox (strict)"("ItemNames"=w507, "ActiveCell"=w502, "CellBG"=w499) -> ()  [unwired: 2 in, 2 out]
        n257 = Increment(x=w497) -> (x+1=w498:i32)
        n258 = Bundle By Name(cluster=w496, "Id"=w498, "Result"=w489) -> (w495:T2)
      }
      frame "Read DF V" {
        # "1.352"
        # "Rounding off to 2 decimal places"
        n259 = Unbundle By Name(w533) -> ("Result"=w528:bool, "Script"=w554:string[][], "Id"=w534:i32)
        n260 = call "ReadFreqVoltage.vi"("channel"=tag "Dev1/ai1") -> ("Ampl"=w530:dbl, "Waveform"=→"DF Voltage":dbl[])  [unwired: 1 in, 8 out]
        n261 = property on="Result" class="MCListbox (strict)"() -> ("ItemNames"=w543:string[][])  [unwired: 2 in, 2 out]
        n262 = Index Array(array=w554, index (row) #1=w534, index (col) #1=3 ("disabled index (col)"), index (row) #2=w534, index (col) #2=2 ("disabled index (col)"), index (row) #3=w534, index (col) #3=1 ("disabled index (col)")) -> (element #1=w550:string, element #2=w549:string, element #3=w548:string)
        n263 = Number To Fractional String(number=w530, precision (6)=i16 2) -> (F-format string=w524:string)  [unwired: 2 out]
        n264 = Fract/Exp String To Number(string=w524) -> (number=w523:dbl)  [unwired: 4 out]
        n265 = Fract/Exp String To Number(string=w549) -> (number=w547:dbl)  [unwired: 4 out]
        n266 = Fract/Exp String To Number(string=w548) -> (number=w546:dbl)  [unwired: 4 out]
        n267 = In Range and Coerce(upper limit=w547, x=w523, lower limit=w546) -> (In Range?=w531:bool)  [unwired: 1 out]
        n268 = Build Array(w550, w549, w548, w524) -> (w545:string[])
        n269 = And(x=w528, y=w531) -> (x .and. y?=w527:bool)
        n270 = Build Array (concatenate)(w556, "Execute Step" ("x")) -> (w555:string[])
        n271 = Array Size(array=w543) -> (size(s)=w542:i32[])
        n272 = Build Array (concatenate)(w543, w545) -> (w544:string[][])
        n273 = Select(t=u32 50176, s=w531, f=u32 12845056) -> (s? t:f=w536:u32)
        n274 = Index Array(array=w542) -> (element=w540:i32)  [unwired: 1 in]
        n275 = Bundle By Name(cluster=T5 {"Row"=-2, "Column"=-2} ("Active Cell:Active Cell"), "Row"=w540) -> (w539:T5)
        n276 = property on="Result" class="MCListbox (strict)"("ItemNames"=w544, "ActiveCell"=w539, "CellBG"=w536) -> ()  [unwired: 2 in, 2 out]
        n277 = Increment(x=w534) -> (x+1=w535:i32)
        n278 = Bundle By Name(cluster=w533, "Id"=w535, "Result"=w527) -> (w532:T2)
      }
      frame "Wait" {
        n279 = Unbundle By Name(w564) -> ("Script"=w568:string[][], "Id"=w565:i32)
        n280 = Index Array(array=w568, index (row)=w565, index (col)=1 ("disabled index (col)")) -> (element=w562:string)
        n281 = Decimal String To Number(string=w562, default (0L)=u32 0 ("default (0 I32)")) -> (number=w561:u32)  [unwired: 2 out]
        n282 = Wait (ms)(milliseconds to wait=w561) -> ()  [unwired: 1 out]
        n283 = Build Array (concatenate)(w570, "Execute Step" ("x")) -> (w569:string[])
        n284 = Increment(x=w565) -> (x+1=w566:i32)
        n285 = Bundle By Name(cluster=w564, "Id"=w566) -> (w563:T2)
      }
      frame "Set Relays" {
        w580 = 4  # index of RunStatus
        n286 = Unbundle By Name(w591) -> ("Script"=w595:string[][], "Id"=w592:i32)
        n287 = Index Array(array=w595, index (row)=w592, index (col)=1 ("disabled index (col)")) -> (element=w589:string)
        n288 = Decimal String To Number(string=w589, default (0L)=u16 0 ("default (0 I32)")) -> (number=w576:u16)  [unwired: 2 out]
        n289 = To Unsigned Word Integer(number=w576) -> (unsigned 16bit integer=w584:u16)
        n290 = Number To Boolean Array(number=w584) -> (Boolean array=w583:bool[])
        n291 = Replace Array Subset(array=w583, new element=TRUE ("new element/subarray"), index=w580) -> (w582:bool[])
        n292 = Boolean Array To Number(Boolean array=w582) -> (number=w581:u32)
        n293 = Build Array (concatenate)(w597, "Execute Step" ("x")) -> (w596:string[])
        n294 = To Unsigned Word Integer(number=w581) -> (unsigned 16bit integer=w578:u16)
        n295 = To Double Precision Float(number=w578) -> (double precision float=w577:dbl)
        n296 = call "EventClient_RaiseEvent.vi"("error in (no error)"=w575, "Data"=w578, "Event"="SetRelays" ("Tag")) -> ("error out"=w574:errorcluster)  [unwired: 1 in, 7 out]
        n297 = call "VariableManager.vi"("Operation"=enum16{"Get Tag", "Set Tag"}."Set Tag", "Value"=w577, "Tag"="RelayOutput") -> ()  [unwired: 9 out]
        n298 = Increment(x=w592) -> (x+1=w593:i32)
        n299 = Bundle By Name(cluster=w591, "Id"=w593) -> (w590:T2)
      }
      frame "Set DO" {
        w612 = 1 items=["one channel for each line", "one channel for all lines"] ("line grouping")
        n300 = Unbundle By Name(w621) -> ("Script"=w624:string[][], "Id"=w603:i32)
        n301 = Index Array(array=w624, index (row) #1=w603, index (col) #1=1 ("disabled index (col)"), index (row) #2=w603, index (col) #2=2 ("index (col)")) -> (element #1=w619:string, element #2=w602:string)
        n302 = Decimal String To Number(string=w619) -> (number=w609:i32)  [unwired: 3 out]
        n303 = Greater Than 0?(x=w609) -> (x > 0?=w608:bool)
        n304 = Select(t=tag "Dev1/port1" ("Port"), s=w608, f=tag "Dev1/port0" ("Port")) -> (s? t:f=w605:tag)
        n305 = Build Array (concatenate)(w626, "Execute Step" ("x")) -> (w625:string[])
        n306 = call-poly <vilib>:"DAQmx Create Virtual Channel.vi"("lines"=w605, "line grouping"=w612, "error in"=w611) -> ("task out"=w614:refnum<k21>, "error out"=w613:errorcluster)  [unwired: 4 in, 7 out]
        n307 = Decimal String To Number(string=w602, default (0L)=u32 0 ("default (0 I32)")) -> (number=w600:u32)  [unwired: 2 out]
        n308 = call <vilib>:"DAQmx Start Task.vi"("task/channels in"=w614, "error in"=w613) -> ("task out"=w616:refnum<k21>, "error out"=w618:errorcluster)  [unwired: 12 out]
        n309 = call-poly <vilib>:"DAQmx Write.vi"("task/channels in"=w616, "data"=w600, "error in"=w618) -> ("task out"=w615:refnum<k21>, "error out"=w617:errorcluster)  [unwired: 1 in, 10 out]
        n310 = call <vilib>:"DAQmx Clear Task.vi"("task in"=w615, "error in"=w617) -> ("error out"=w610:errorcluster)  [unwired: 13 out]
        n311 = Increment(x=w603) -> (x+1=w622:i32)
        n312 = Bundle By Name(cluster=w621, "Id"=w622) -> (w620:T2)
      }
      frame "Refresh Sr Nos" {
        n313 = Unbundle By Name(w636) -> ("WORef"=w638:T1)
        n314 = call "WorkorderHandler_LatestSr.vi"("error in (no error)"=w631, "reference"=w638) -> ("error out"=w630:errorcluster, "Bad"=w633:string, "OK"=w635:string, "SrNo"=w637:string)  [unwired: 6 out]
        n315 = Decimal String To Number(string=w635) -> (number=w634:i32)  [unwired: 3 out]
        n316 = Decimal String To Number(string=w633) -> (number=w632:i32)  [unwired: 3 out]
        n317 = local write "Part Number"(w637) -> ()
        n318 = local write "Good Boards"(w634) -> ()
        n319 = local write "Bad Boards"(w632) -> ()
      }
      frame "Set Load" {
        n320 = Unbundle By Name(w644) -> ("Script"=w654:string[][], "Id"=w641:i32)
        n321 = Index Array(array=w654, index (row) #1=w641, index (col) #1=1 ("disabled index (col)"), index (row) #2=w641, index (col) #2=2 ("disabled index (col)")) -> (element #1=w651:string)  [unwired: 1 out]
        n322 = Decimal String To Number(string=w651, default (0L)=u8 0 ("default (0 I32)")) -> (number=w640:u8)  [unwired: 1 in, 1 out]
        n323 = disable-structure shown="Enabled" {
          disable-tunnel: w649 -> [w670 w674]
          disable-tunnel: [w666 w673] -> w648
          disable-tunnel: w640 -> [w656 w675]
          frame Disabled {
            n324 = call "SerialSettings.vi"("Operation"=Settings_Operation."Get Value", "error in (no error)"=w670) -> ("error out"=w669:errorcluster, "Serial Info Out"=w671:T9)  [unwired: 8 in]
            n325 = Unbundle By Name(w671) -> ("Port"=w663:refnum<visa-resource-name>, "baud rate"=w662:u32, "data bits"=w661:u16, "parity"=w660:enum16{"None", "Odd", "Even", "Mark", "Space"}, "stop bits"=w659:u16, "flow control"=w658:u16)
            n326 = call-poly "VISA Configure Serial Port"("VISA resource name"=w663, "baud rate (9600)"=w662, "data bits (8)"=w661, "parity (0:none)"=w660, "error in (no error)"=w669, "stop bits (10: 1 bit)"=w659, "flow control (0:none)"=w658) -> ("VISA resource name out"=w665:refnum<visa-resource-name>, "error out"=w668:errorcluster)  [unwired: 7 in]
            n327 = Number To Decimal String(number=w656) -> (decimal integer string=w657:string)  [unwired: 1 in]
            n328 = VISA Write(VISA resource name=w665, write buffer=w657, error in (no error)=w668) -> (VISA resource name out=w664:refnum<visa-resource-name>, error out=w667:errorcluster)  [unwired: 1 out]
            n329 = VISA Close(VISA resource name=w664, error in (no error)=w667) -> (error out=w666:errorcluster)
          }
          frame Enabled {
            n330 = call "EventClient_RaiseEvent.vi"("error in (no error)"=w674, "Data"=w675, "Event"="SetLoad") -> ("error out"=w673:errorcluster)  [unwired: 1 in, 7 out]
          }
        }
        n331 = Build Array (concatenate)(w646, "Execute Step" ("x")) -> (w645:string[])
        n332 = Increment(x=w641) -> (x+1=w642:i32)
        n333 = Bundle By Name(cluster=w644, "Id"=w642) -> (w643:T2)
      }
      frame "---------------Below are Error Handling VIs---------------" {
        # "This State will never Execute\nIt is added just for improving code readability please do not remove this case"
      }
      frame "Error" {
      }
    }
    n334 = call "Error Handler.vi"("Current State"=w14, "error in (no error)"=w12, "Msg Queue In"=w15) -> ("error out"=w13:errorcluster, "Msg Queue Out"=w16:string[])  [unwired: 7 out]
  }
  n335 = property class="App"(error in=w2) -> (error out=→"error out":errorcluster, "App.Kind"=w5:T3)  [unwired: 1 in, 1 out]
  n336 = Equal?(x=w5, y=T3."Run Time System" ("Application:Kind")) -> (x = y?=w3:bool)
  n337 = Quit LabVIEW(quit? (T)=w3) -> ()
